vi "Old Limits Page.vi"(8 "error in (no error)":errorcluster, 10 "LBCB Number":T2) -> (0 "error out":errorcluster)   [LabVIEW 2013]
uses:
  lib/Limits/Faults List Actions.ctl
  lib/Limits Widget/Lower Upper Select.ctl
  lib/Limits Widget/Slider Messages.ctl
  lib/Data Access Objects/Metadata/LBCB Number.ctl
  lib/Control Loop/Parameter Change States.ctl
  lib/Control Loop/Parameters Changes.ctl
  lib/Data Access Objects/Application/Number Of LBCBs.ctl
  lib/Data Access Objects/Metadata/Persistant DAO Actions.ctl
  lib/Launcher/Launcher Actions.ctl
  lib/Launcher/NoPanelAppTypes.ctl
  lib/Logging/Debug Type.ctl
  lib/Limits Widget/Limits Page Visible Elements.ctl
  lib/Limits Widget/Limit Slider.ctl
  lib/Data Access Objects/Limits/DofTypes.ctl
panel:
  out "Messages":string
  in  "Ok":bool
  in  "DofType":T1
  in  "Limit Slider 6":T3
  in  "Limit Slider 5":T3
  in  "Limit Slider 4":T3
  in  "Limit Slider 3":T3
  in  "Limit Slider 2":T3
  in  "Limit Slider 1":T3
  # "Lower"
  # "Higher"
  # "Current"
  # "Lower"
  # "Higher"
  # "Current"
  # "Global"
  # "Local"
  # "Lower"
  # "Higher"
  # "Current"
  # "Lower"
  # "Higher"
  # "Current"
  # "Global"
  # "Local"
  # "Lower"
  # "Higher"
  # "Current"
  # "Lower"
  # "Higher"
  # "Current"
  # "Global"
  # "Local"
  # "Lower"
  # "Higher"
  # "Current"
  # "Lower"
  # "Higher"
  # "Current"
  # "Global"
  # "Local"
  # "Lower"
  # "Higher"
  # "Current"
  # "Lower"
  # "Higher"
  # "Current"
  # "Global"
  # "Local"
  # "Lower"
  # "Higher"
  # "Current"
  # "Lower"
  # "Higher"
  # "Current"
  # "Global"
  # "Local"
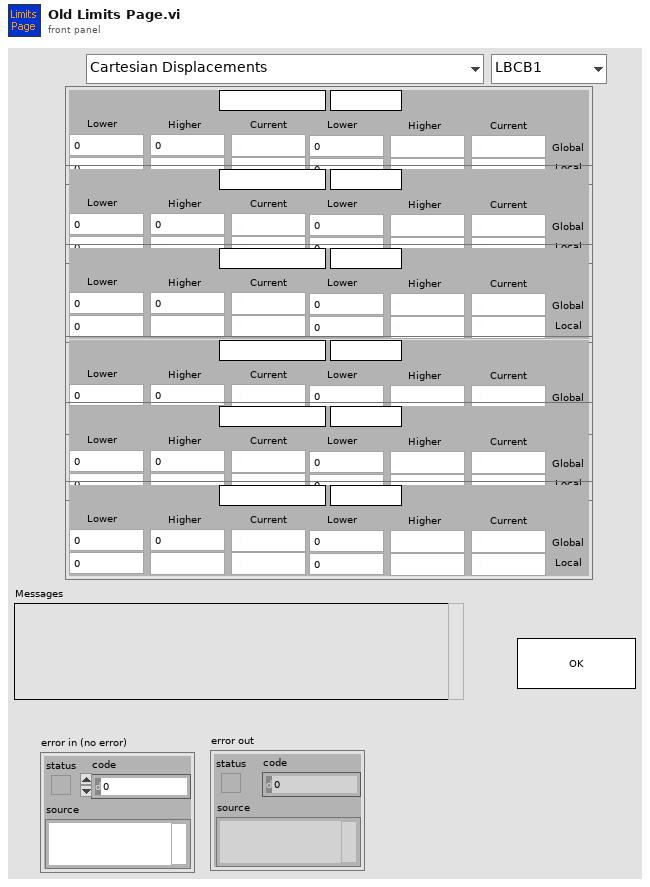
[diagram p1: front panel]
types:
  T1 = typedef "DofTypes.ctl" = enum16{"Cartesian Displacements", "Cartesian Forces & Moments", "Actuator Displacements", "Actuator Forces", "Cartesian Increments", "Actuator Increments"}
  T2 = typedef "LBCB Number.ctl" = enum16{"LBCB1", "LBCB2"}
  T3 = typedef "Limit Slider.ctl" = cluster{"DofLabel":string, "Units":string, "Global Lo 1":dbl, "Local Lo 1":dbl, "Global Hi 1":dbl, "Local Hi 1":dbl, "Global Actual 1":dbl, "Local Actual 1":dbl, "Global Lo 2":dbl, "Local Lo 2":dbl, "Global Hi 2":dbl, "Global Actual 2":dbl, "Local Hi 2":dbl, "Local Actual 2":dbl}
  T4 = typedef "Parameters Changes.ctl" = cluster{"Change State":T5, "LBCB Number":T2}
  T5 = typedef "Parameter Change States.ctl" = enum16{"Mixed Mode", "Control Loop", "Limits", "Application", "Stiffness Jacobian", "Start DAQ", "Reset Auto-Balance", "Set Command", "Enable Control", "Disable Control", "Position", "Stop Application"}
  T6 = typedef "Slider Messages.ctl" = enum16{"Update Display", "Exit", "Nothing"}
  T7 = typedef "Persistant DAO Actions.ctl" = enum16{"Init", "Get", "Set", "Load", "Save"}
  T8 = enum8{"Enabled", "Disabled", "Disabled and Grayed Out"}
  T9 = typedef "Number Of LBCBs.ctl" = enum16{"1", "2"}
  T10 = typedef "Faults List Actions.ctl" = enum16{"Init", "Add", "Remove", "Get List"}
  T11 = typedef "Lower Upper Select.ctl" = enum16{"Lower", "Upper"}
  T12 = typedef "Debug Type.ctl" = enum16{"Limit Update", "Limit Change", ""}
  T13 = typedef "Limits Page Visible Elements.ctl" = enum16{"All", "Global Only", "Low Only"}
  T14 = typedef "Fault Id.ctl" = cluster{"Fault Type":T15, "LBCB Number":T2, "Index":u32, "Space Type":T16}
  T15 = typedef "Fault Type.ctl" = enum16{"None", "Command", "Displacement", "Force", "Increment"}
  T16 = typedef "Space Type.ctl" = enum16{"Actuator", "Cartesian"}
  T17 = cluster{"[0]":dbl, "[1]":dbl, "[2]":dbl, "[3]":dbl, "[4]":dbl, "[5]":dbl, "[6]":dbl, "[7]":dbl, "[8]":dbl}[]
  T18 = cluster{"[0]":dbl, "[1]":dbl, "[2]":dbl, "[3]":dbl, "[4]":dbl, "[5]":dbl, "[6]":dbl, "[7]":dbl, "[8]":dbl}
  T19 = cluster{"[0]":dbl, "[1]":dbl, "[2]":dbl, "[3]":dbl}
  T20 = typedef "NoPanelAppTypes.ctl" = enum16{"NTCP Socket", "Data Archiving", "DAQ Link", "Control Loops", "Cmd Disp Diffs", "LBCB Data", "Limits", "Mixed Mode Widget", "Offsets", "Debug"}
  T21 = typedef "Launcher Actions.ctl" = enum16{"Launch", "Stop All", "Stop", "Kill", "Running?", "Init"}
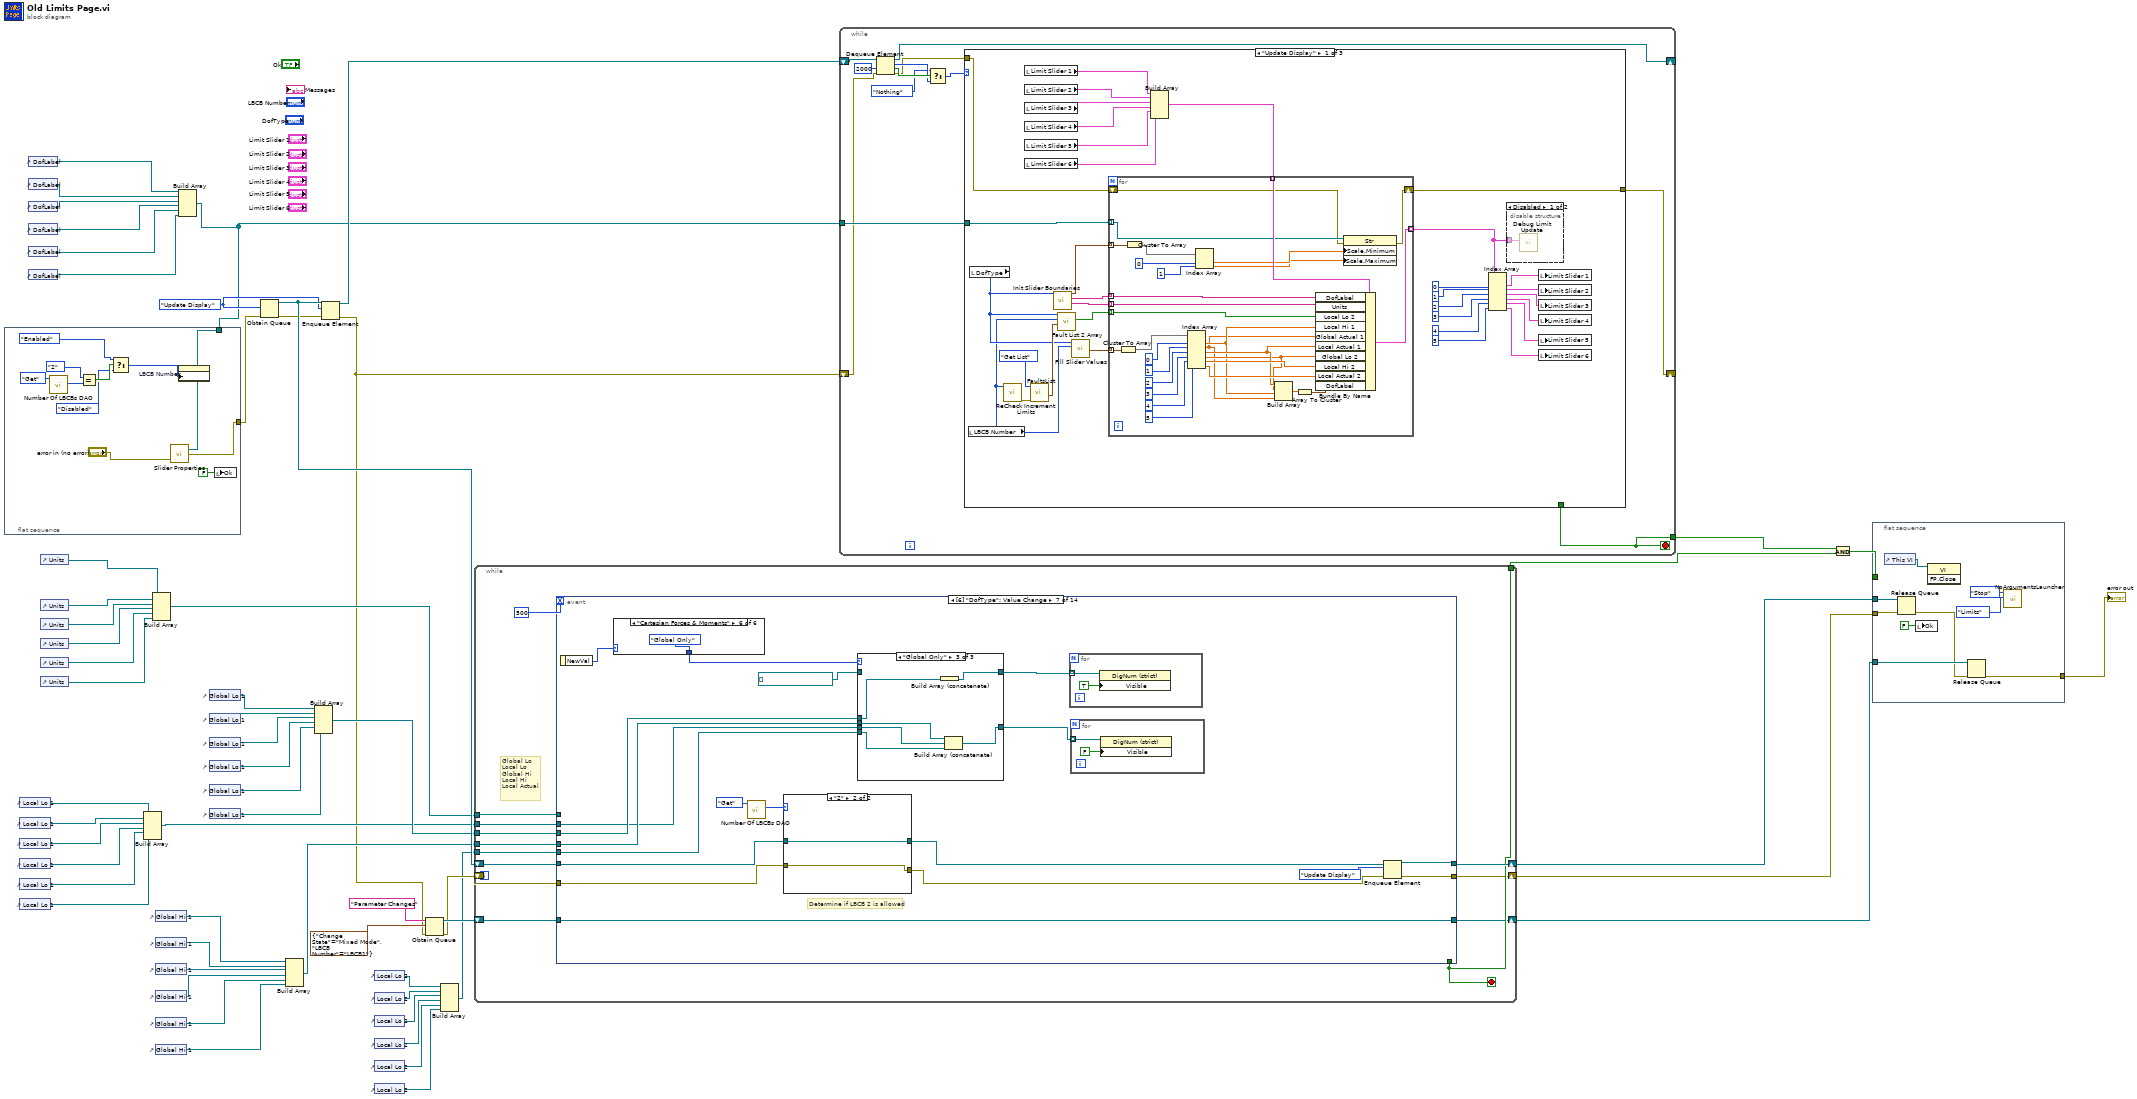
[diagram p0: block diagram]
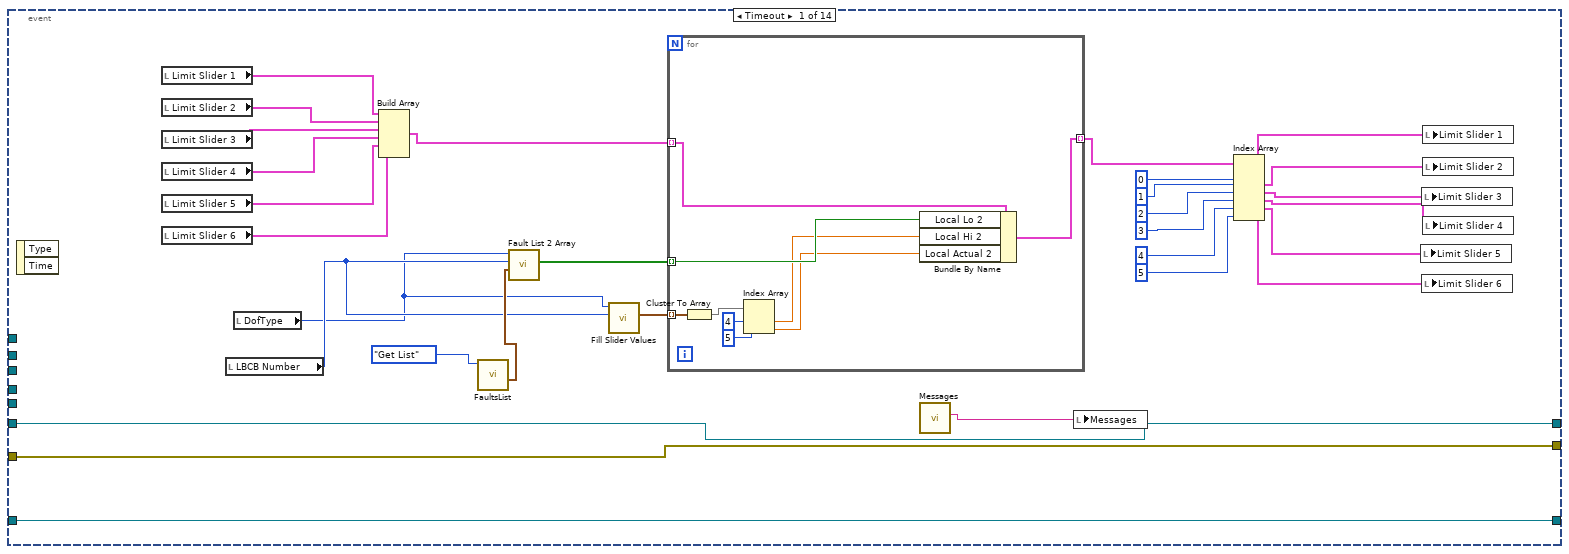
[diagram p2: hidden frame]
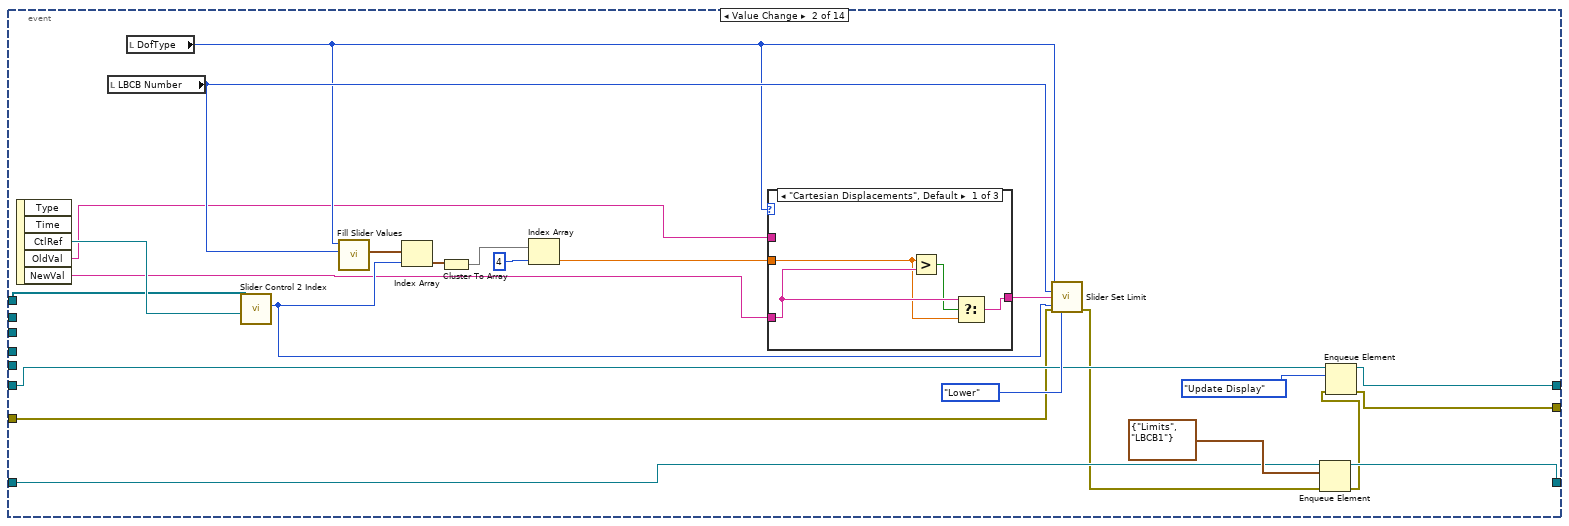
[diagram p3: hidden frame]
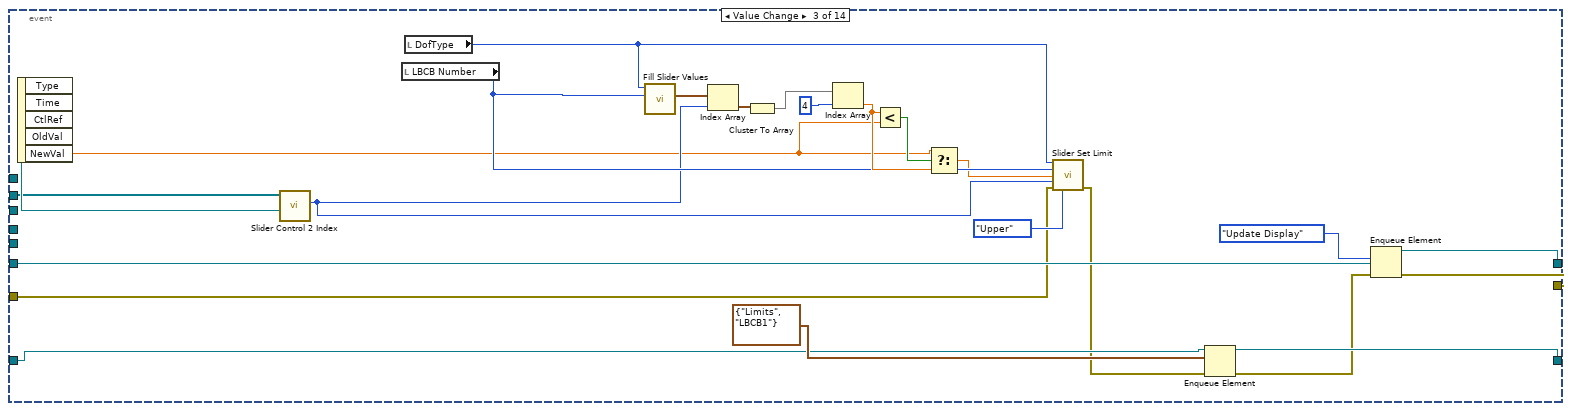
[diagram p6: hidden frame]
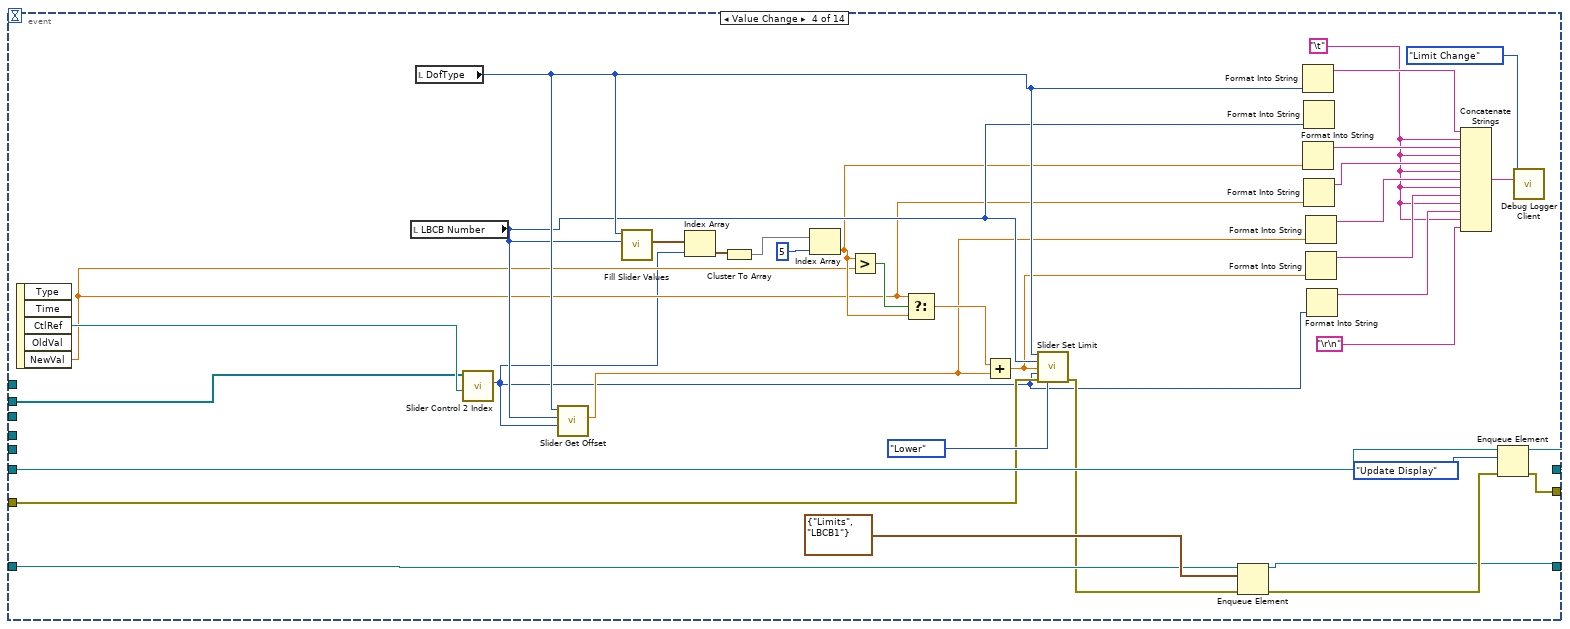
[diagram p7: hidden frame]
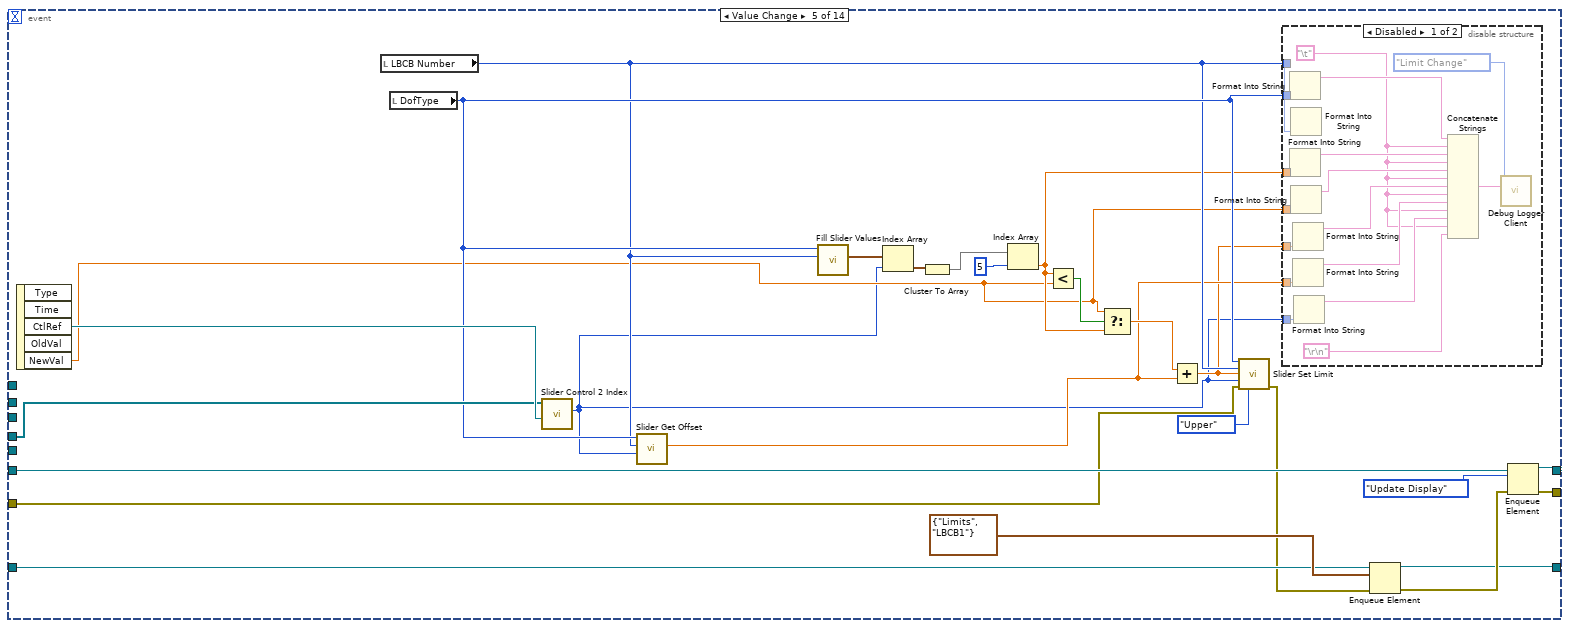
[diagram p8: hidden frame]
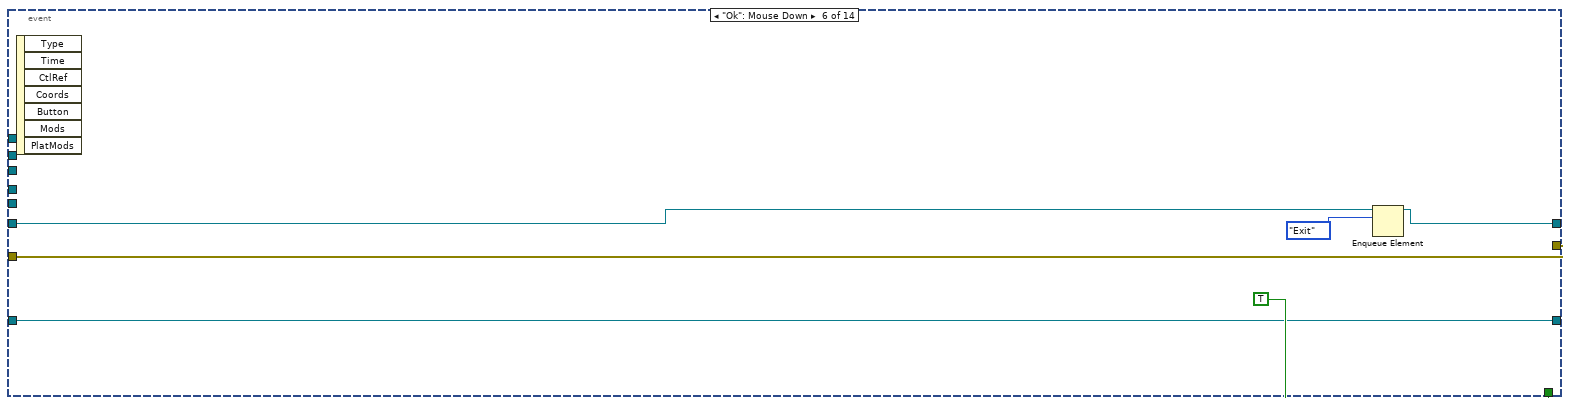
[diagram p10: hidden frame]
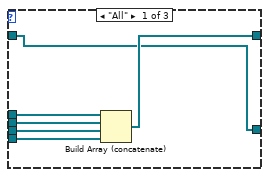
[diagram p11: hidden frame]
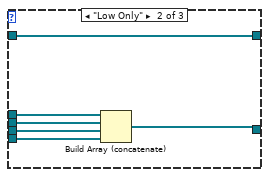
[diagram p12: hidden frame]
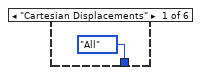
[diagram p13: hidden frame]
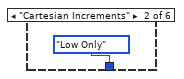
[diagram p14: hidden frame]
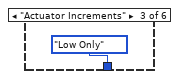
[diagram p15: hidden frame]
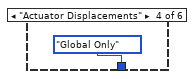
[diagram p16: hidden frame]
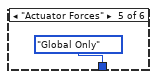
[diagram p17: hidden frame]
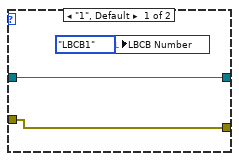
[diagram p18: hidden frame]
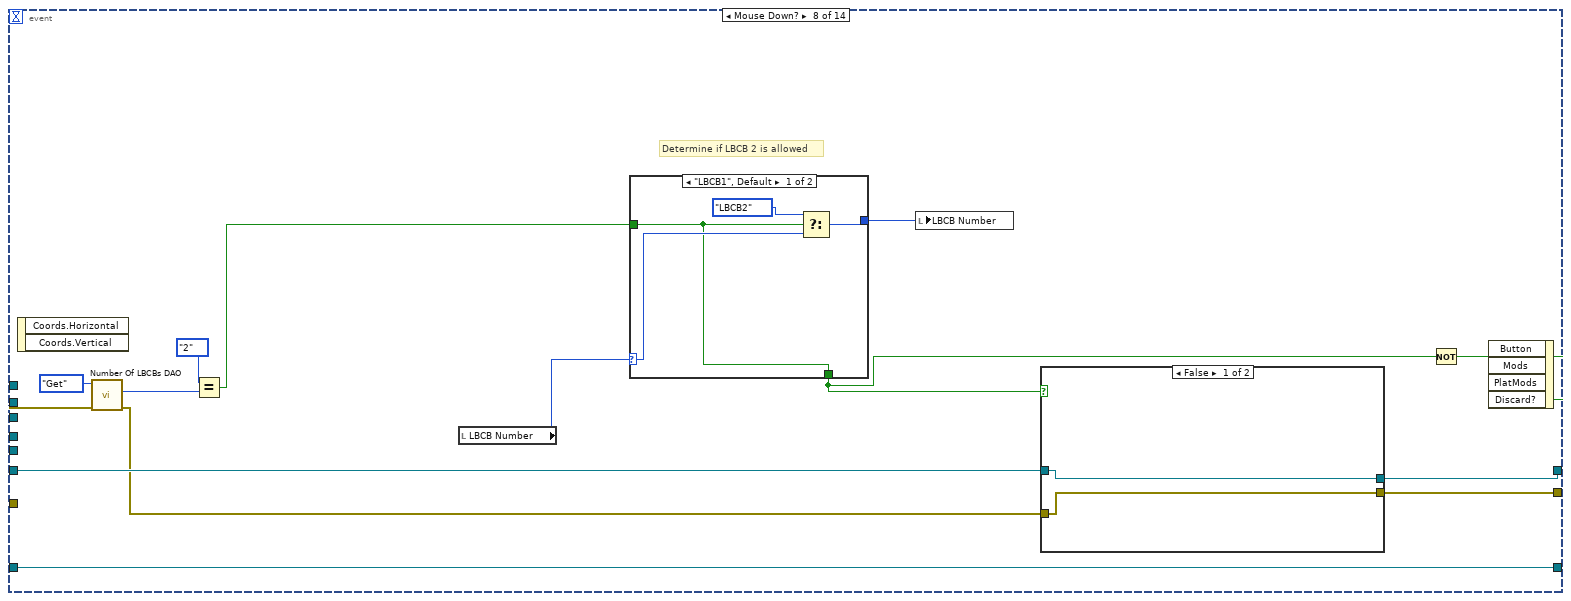
[diagram p19: hidden frame]
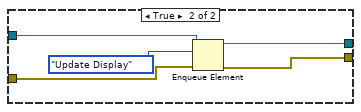
[diagram p20: hidden frame]
diagram:
  w54 = Slider_Messages."Update Display" ("Slider Message")
  n1 = flat-sequence {
    tunnel: w19 -> [w69]
    tunnel: [w68] -> w18
    frame #0 {
      n2 = call "Number Of LBCBs DAO.vi"("Actions"=Persistant_DAO_Actions."Get") -> ("Number of\nLBCBs Out"=w67:T9)  [unwired: 7 in, 3 out]
      n3 = Equal?(x=Number_Of_LBCBs."2", y=w67) -> (x = y?=w65:bool)
      n4 = Select(t=T8."Enabled" ("Disabled"), s=w65, f=T8."Disabled") -> (s? t:f=w62:T8)
      n5 = call "Slider Properties.vi"("error in (no error) 2"="error in (no error)", "Array"=w69) -> ("error out"=w68:errorcluster)
      n6 = property on="LBCB Number" class="Enum (strict)"("DisabledEnum"=w62) -> ()  [unwired: 2 in, 2 out]
      n7 = local write "Ok"(FALSE ("Ok")) -> ()
    }
  }
  n8 = control-ref of="Local Lo 1"() -> (w41:refnum<vi>)
  n9 = control-ref of="Local Lo 1"() -> (w40:refnum<vi>)
  n10 = control-ref of="Local Lo 1"() -> (w39:refnum<vi>)
  n11 = control-ref of="Local Lo 1"() -> (w38:refnum<vi>)
  n12 = control-ref of="Local Lo 1"() -> (w37:refnum<vi>)
  n13 = control-ref of="Local Lo 1"() -> (w36:refnum<vi>)
  n14 = control-ref of="DofLabel"() -> (w53:refnum<vi>)
  n15 = control-ref of="DofLabel"() -> (w52:refnum<vi>)
  n16 = control-ref of="DofLabel"() -> (w51:refnum<vi>)
  n17 = control-ref of="DofLabel"() -> (w50:refnum<vi>)
  n18 = control-ref of="DofLabel"() -> (w49:refnum<vi>)
  n19 = control-ref of="DofLabel"() -> (w48:refnum<vi>)
  n20 = control-ref of="Units"() -> (w47:refnum<vi>)
  n21 = control-ref of="Units"() -> (w46:refnum<vi>)
  n22 = control-ref of="Units"() -> (w45:refnum<vi>)
  n23 = control-ref of="Units"() -> (w44:refnum<vi>)
  n24 = control-ref of="Units"() -> (w43:refnum<vi>)
  n25 = control-ref of="Units"() -> (w42:refnum<vi>)
  n26 = Build Array(w41, w40, w39, w38, w37, w36) -> (w22:refnum<vi>[])
  n27 = Build Array(w47, w46, w45, w44, w43, w42) -> (w21:refnum<vi>[])
  n28 = control-ref of="Global Hi 1"() -> (w29:refnum<vi>)
  n29 = control-ref of="Global Hi 1"() -> (w28:refnum<vi>)
  n30 = control-ref of="Global Hi 1"() -> (w16:refnum<vi>)
  n31 = control-ref of="Global Hi 1"() -> (w27:refnum<vi>)
  n32 = control-ref of="Global Hi 1"() -> (w26:refnum<vi>)
  n33 = control-ref of="Global Hi 1"() -> (w25:refnum<vi>)
  n34 = Build Array(w53, w52, w51, w50, w49, w48) -> (w19:refnum<vi>[])
  n35 = control-ref of="Global Lo 1"() -> (w35:refnum<vi>)
  n36 = control-ref of="Global Lo 1"() -> (w34:refnum<vi>)
  n37 = control-ref of="Global Lo 1"() -> (w33:refnum<vi>)
  n38 = control-ref of="Global Lo 1"() -> (w32:refnum<vi>)
  n39 = control-ref of="Global Lo 1"() -> (w31:refnum<vi>)
  n40 = control-ref of="Global Lo 1"() -> (w30:refnum<vi>)
  n41 = Obtain Queue(element data type=w54, error in (no error)=w18) -> (queue out=w59:refnum<queue>, error out=w20:errorcluster)  [unwired: 3 in, 1 out]
  n42 = Build Array(w29, w28, w16, w27, w26, w25) -> (w24:refnum<vi>[])
  n43 = Build Array(w35, w34, w33, w32, w31, w30) -> (w23:refnum<vi>[])
  n44 = Enqueue Element(queue=w59, element=w54, error in (no error)=w20) -> (queue out=w55:refnum<queue>, error out=w12:errorcluster)  [unwired: 1 in, 1 out]
  n45 = control-ref of="Local Lo 2"() -> (w7:refnum<vi>)
  n46 = control-ref of="Local Lo 2"() -> (w6:refnum<vi>)
  n47 = control-ref of="Local Lo 2"() -> (w5:refnum<vi>)
  n48 = control-ref of="Local Lo 2"() -> (w4:refnum<vi>)
  n49 = control-ref of="Local Lo 2"() -> (w3:refnum<vi>)
  n50 = control-ref of="Local Lo 2"() -> (w2:refnum<vi>)
  n51 = Obtain Queue(name (unnamed)="Parameter Changes", element data type=T4 {"Change State"=enum."Mixed Mode", "LBCB Number"=enum."LBCB1"} ("Parameter Changes"), error in (no error)=w12) -> (queue out=w13:refnum<queue>, error out=w11:errorcluster)  [unwired: 2 in, 1 out]
  n52 = Build Array(w7, w6, w5, w4, w3, w2) -> (w1:refnum<vi>[])
  n53 = while {
    shift-right: [w82] -> w17
    shift-left: w59 -> [w83]
    tunnel: [w81] -> w57
    tunnel: w24 -> [w78]
    tunnel: w23 -> [w77]
    tunnel: w22 -> [w79]
    tunnel: w21 -> [w80]
    shift-right: [w75] -> w9
    shift-left: w11 -> [w76]
    shift-right: [w73] -> w10
    shift-left: w13 -> [w74]
    tunnel: w1 -> [w72]
    stop <- w81 stop-if-true
    # "Global Lo\nLocal Lo\nGlobal Hi\nLocal Hi\nLocal Actual"
    n54 = event shown="[6] \"DofType\": Value Change" {
      selector: _ -> [_ _ _ _ _ _ _ _ _ _ _ _ _ _]
      dyn-events: _ -> [_ _ _ _ _ _ _ _ _ _ _ _ _ _]
      timeout: 500 -> [_ _ _ _ _ _ _ _ _ _ _ _ _ _]
      tunnel: w83 -> [w112 w143 w173 w209 w236 w260 w275 w327 w348 w397 w446 w497 w544 w593]
      tunnel: [w112 w142 w172 w208 w234 w259 w279 w326 w347 w396 w445 w496 w543 w592] -> w82
      tunnel: [_ _ _ _ _ TRUE _ _ _ _ _ _ _ _] -> w81
      tunnel: w80 -> [_ w141 _ _ _ _ _ _ _ _ _ _ _ _]
      tunnel: w79 -> [_ _ _ w207 _ _ w266 _ _ _ _ _ _ _]
      tunnel: w78 -> [_ _ _ _ w233 _ w268 _ _ _ _ _ _ _]
      tunnel: w77 -> [_ _ w171 _ _ _ w269 _ _ _ _ _ _ _]
      tunnel: w76 -> [w111 w140 w170 w206 w232 w257 w273 w323 w350 w399 w448 w499 w546 w595]
      tunnel: [w111 w139 w169 w205 w231 w257 w278 w325 w346 w395 w444 w495 w542 w591] -> w75
      tunnel: w74 -> [w110 w137 w167 w203 w229 w256 w277 w324 w344 w393 w442 w491 w540 w589]
      tunnel: [w110 w136 w166 w200 w226 w256 w277 w324 w343 w392 w440 w490 w539 w588] -> w73
      tunnel: w72 -> [_ _ _ _ _ _ w265 _ _ _ _ _ _ _]
      event Timeout {
        n55 = event-data() -> ()  [unwired: 1 in, 2 out]
        n56 = local read "Limit Slider 1"() -> (w107:T3)
        n57 = local read "Limit Slider 2"() -> (w106:T3)
        n58 = local read "Limit Slider 3"() -> (w105:T3)
        n59 = local read "Limit Slider 4"() -> (w104:T3)
        n60 = local read "Limit Slider 5"() -> (w103:T3)
        n61 = local read "Limit Slider 6"() -> (w102:T3)
        n62 = local read "LBCB Number"() -> (w86:T2)
        n63 = local read "DofType"() -> (w85:T1)
        n64 = Build Array(w107, w106, w105, w104, w103, w102) -> (w94:T3[])
        n65 = call "FaultsList.vi"("Limits List Actions"=Faults_List_Actions."Get List") -> ("Fault List"=w108:T14[])  [unwired: 2 in, 8 out]
        n66 = call "Fault List 2 Array.vi"("Fault List"=w108, "LBCB Number"=w86, "DofType"=w85) -> ("Faults"=w95:bool[])  [unwired: 8 in]
        n67 = call "Fill Slider Values.vi"("LBCB Number"=w86, "DofType"=w85) -> ("Silder Values"=w84:T17)  [unwired: 9 in]
        n68 = for {
          tunnel: w95 -> [w121] mode=indexing
          tunnel: w94 -> [w122] mode=indexing
          tunnel: [w120] -> w93 mode=indexing
          tunnel: w84 -> [w119] mode=indexing
          n69 = Cluster To Array(cluster=w119) -> (array=w118:dbl[])
          n70 = Index Array(array=w118, index #1=4 ("index"), index #2=5 ("index")) -> (element #1=w115:dbl, element #2=w114:dbl)
          n71 = Bundle By Name(cluster=w122, "Local Lo 2"=w121, "Local Hi 2"=w115, "Local Actual 2"=w114) -> (w120:T3)
        }
        n72 = call "Messages.vi"() -> ("Messages"=w113:string)  [unwired: 2 in, 9 out]
        n73 = local write "Messages"(w113) -> ()
        n74 = Index Array(array=w93, index #1=0 ("index"), index #2=1 ("index"), index #3=2 ("index"), index #4=3 ("index"), index #5=4 ("index"), index #6=5 ("index")) -> (element #1=w92:T3, element #2=w91:T3, element #3=w90:T3, element #4=w89:T3, element #5=w88:T3, element #6=w87:T3)
        n75 = local write "Limit Slider 5"(w88) -> ()
        n76 = local write "Limit Slider 3"(w90) -> ()
        n77 = local write "Limit Slider 6"(w87) -> ()
        n78 = local write "Limit Slider 1"(w92) -> ()
        n79 = local write "Limit Slider 2"(w91) -> ()
        n80 = local write "Limit Slider 4"(w89) -> ()
      }
      event Value Change {
        n81 = event-data() -> ("CtlRef"=w146:refnum<vi>, "OldVal"=w123:string, "NewVal"=w127:string)  [unwired: 1 in, 2 out]
        n82 = local read "LBCB Number"() -> (w133:T2)
        n83 = local read "DofType"() -> (w124:T1)
        n84 = call "Slider Control 2 Index.vi"("Control"=w146, "Controls"=w141) -> ("Index"=w131:i32)  [unwired: 9 in]
        n85 = call "Fill Slider Values.vi"("LBCB Number"=w133, "DofType"=w124) -> ("Silder Values"=w132:T17)  [unwired: 9 in]
        n86 = Index Array(array=w132, index=w131) -> (element=w130:T18)
        n87 = Cluster To Array(cluster=w130) -> (array=w129:dbl[])
        n88 = Index Array(array=w129, index=4) -> (element=w125:dbl)
        n89 = case shown="\"Cartesian Displacements\", Default" w124 {
          tunnel: w127 -> [w150 w151 w152]
          tunnel: [w149 w151 w152] -> w126
          tunnel: w125 -> [w147 _ _]
          tunnel: w123 -> [_ _ _]
          frame "Cartesian Displacements", Default {
            n90 = Greater?(x=w147, y=w150) -> (0:w148:bool)
            n91 = Select(t=w150, s=w148, f=w147) -> (s? t:f=w149:string)
          }
          frame "Cartesian Increments" {
          }
          frame "Actuator Increments" {
          }
        }
        n92 = call "Slider Set Limit.vi"("DofType"=w124, "LBCB Number"=w133, "Value"=w126, "Index"=w131, "error in (no error)"=w140, "Lower/Upper"=Lower_Upper_Select."Lower") -> ("error out"=w135:errorcluster)  [unwired: 9 in]
        n93 = Enqueue Element(queue=w137, element=T4 {"Change State"=enum."Limits", "LBCB Number"=enum."LBCB1"}, error in (no error)=w135) -> (queue out=w136:refnum<queue>, error out=w134:errorcluster)  [unwired: 2 out]
        n94 = Enqueue Element(queue=w143, element=Slider_Messages."Update Display", error in (no error)=w134) -> (queue out=w142:refnum<queue>, error out=w139:errorcluster)  [unwired: 1 in, 1 out]
      }
      event Value Change {
        n95 = event-data() -> ("CtlRef"=w176:refnum<vi>, "NewVal"=w153:dbl)  [unwired: 1 in, 3 out]
        n96 = call "Slider Control 2 Index.vi"("Control"=w176, "Controls"=w171) -> ("Index"=w155:i32)  [unwired: 9 in]
        n97 = local read "LBCB Number"() -> (w156:T2)
        n98 = local read "DofType"() -> (w157:T1)
        n99 = call "Fill Slider Values.vi"("LBCB Number"=w156, "DofType"=w157) -> ("Silder Values"=w163:T17)  [unwired: 9 in]
        n100 = Index Array(array=w163, index=w155) -> (element=w162:T18)
        n101 = Cluster To Array(cluster=w162) -> (array=w161:dbl[])
        n102 = Index Array(array=w161, index=4) -> (element=w158:dbl)
        n103 = Less?(x=w158, y=w153) -> (x < y?=w159:bool)
        n104 = Select(t=w153, s=w159, f=w158) -> (s? t:f=w154:dbl)
        n105 = call "Slider Set Limit.vi"("DofType"=w157, "LBCB Number"=w156, "Value"=w154, "Index"=w155, "error in (no error)"=w170, "Lower/Upper"=Lower_Upper_Select."Upper") -> ("error out"=w165:errorcluster)  [unwired: 9 in]
        n106 = Enqueue Element(queue=w167, element=T4 {"Change State"=enum."Limits", "LBCB Number"=enum."LBCB1"}, error in (no error)=w165) -> (queue out=w166:refnum<queue>, error out=w164:errorcluster)  [unwired: 2 out]
        n107 = Enqueue Element(queue=w173, element=Slider_Messages."Update Display", error in (no error)=w164) -> (queue out=w172:refnum<queue>, error out=w169:errorcluster)  [unwired: 1 in, 1 out]
      }
      event Value Change {
        w187 = "\t"
        n108 = event-data() -> ("CtlRef"=w212:refnum<vi>, "NewVal"=w180:dbl)  [unwired: 1 in, 3 out]
        n109 = local read "LBCB Number"() -> (w182:T2)
        n110 = local read "DofType"() -> (w183:T1)
        n111 = call "Slider Control 2 Index.vi"("Control"=w212, "Controls"=w207) -> ("Index"=w177:i32)  [unwired: 9 in]
        n112 = call "Slider Get Offset.vi"("Index"=w177, "LBCB Number"=w182, "DofType"=w183) -> ("Offset"=w179:dbl)  [unwired: 8 in]
        n113 = call "Fill Slider Values.vi"("LBCB Number"=w182, "DofType"=w183) -> ("Silder Values"=w199:T17)  [unwired: 9 in]
        n114 = Index Array(array=w199, index=w177) -> (element=w198:T18)
        n115 = Cluster To Array(cluster=w198) -> (array=w197:dbl[])
        n116 = Index Array(array=w197, index=5) -> (element=w181:dbl)
        n117 = Greater?(x=w181, y=w180) -> (0:w195:bool)
        n118 = Select(t=w180, s=w195, f=w181) -> (s? t:f=w194:dbl)
        n119 = Add(x=w194, y=w179) -> (x+y=w178:dbl)
        n120 = call "Slider Set Limit.vi"("DofType"=w183, "LBCB Number"=w182, "Value"=w178, "Index"=w177, "error in (no error)"=w206, "Lower/Upper"=Lower_Upper_Select."Lower") -> ("error out"=w202:errorcluster)  [unwired: 9 in]
        n121 = Enqueue Element(queue=w203, element=T4 {"Change State"=enum."Limits", "LBCB Number"=enum."LBCB1"}, error in (no error)=w202) -> (queue out=w200:refnum<queue>, error out=w201:errorcluster)  [unwired: 2 out]
        n122 = Format Into String(w183) -> (resulting string=w193:string)  [unwired: 3 in, 1 out]
        n123 = Format Into String(w181) -> (resulting string=w192:string)  [unwired: 3 in, 1 out]
        n124 = Format Into String(w182) -> ()  [unwired: 3 in, 2 out]
        n125 = Format Into String(w180) -> (resulting string=w191:string)  [unwired: 3 in, 1 out]
        n126 = Format Into String(w179) -> (resulting string=w190:string)  [unwired: 3 in, 1 out]
        n127 = Format Into String(w178) -> (resulting string=w189:string)  [unwired: 3 in, 1 out]
        n128 = Format Into String(w177) -> (resulting string=w188:string)  [unwired: 3 in, 1 out]
        n129 = Concatenate Strings(w193, w187, w192, w187, w191, w187, w190, w187, w189, w187, w188, w187, "\r\n") -> (w185:string)
        n130 = Enqueue Element(queue=w209, element=Slider_Messages."Update Display", error in (no error)=w201) -> (queue out=w208:refnum<queue>, error out=w205:errorcluster)  [unwired: 1 in, 1 out]
        n131 = call "Debug Logger Client.vi"("Message"=w185, "Debug Type"=Debug_Type."Limit Change") -> ()  [unwired: 9 in, 1 out]
      }
      event Value Change {
        n132 = event-data() -> ("CtlRef"=w238:refnum<vi>, "NewVal"=w217:dbl)  [unwired: 1 in, 3 out]
        n133 = local read "LBCB Number"() -> (w219:T2)
        n134 = local read "DofType"() -> (w220:T1)
        n135 = call "Slider Control 2 Index.vi"("Control"=w238, "Controls"=w233) -> ("Index"=w213:i32)  [unwired: 9 in]
        n136 = call "Slider Get Offset.vi"("Index"=w213, "LBCB Number"=w219, "DofType"=w220) -> ("Offset"=w215:dbl)  [unwired: 8 in]
        n137 = call "Fill Slider Values.vi"("LBCB Number"=w219, "DofType"=w220) -> ("Silder Values"=w225:T17)  [unwired: 9 in]
        n138 = Index Array(array=w225, index=w213) -> (element=w224:T18)
        n139 = Cluster To Array(cluster=w224) -> (array=w223:dbl[])
        n140 = Index Array(array=w223, index=5) -> (element=w218:dbl)
        n141 = Less?(x=w218, y=w217) -> (x < y?=w221:bool)
        n142 = Select(t=w217, s=w221, f=w218) -> (s? t:f=w216:dbl)
        n143 = Add(x=w216, y=w215) -> (x+y=w214:dbl)
        n144 = call "Slider Set Limit.vi"("DofType"=w220, "LBCB Number"=w219, "Value"=w214, "Index"=w213, "error in (no error)"=w232, "Lower/Upper"=Lower_Upper_Select."Upper") -> ("error out"=w228:errorcluster)  [unwired: 9 in]
        n145 = disable-structure shown="Disabled" {
          disable-tunnel: w220 -> [w255 _]
          disable-tunnel: w219 -> [w254 _]
          disable-tunnel: w218 -> [w253 _]
          disable-tunnel: w217 -> [w252 _]
          disable-tunnel: w215 -> [w251 _]
          disable-tunnel: w214 -> [w250 _]
          disable-tunnel: w213 -> [w249 _]
          frame Disabled {
            w242 = "\t"
            n146 = Format Into String(w255) -> (resulting string=w248:string)  [unwired: 3 in, 1 out]
            n147 = Format Into String(w253) -> (resulting string=w247:string)  [unwired: 3 in, 1 out]
            n148 = Format Into String(w254) -> ()  [unwired: 3 in, 2 out]
            n149 = Format Into String(w252) -> (resulting string=w246:string)  [unwired: 3 in, 1 out]
            n150 = Format Into String(w250) -> (resulting string=w245:string)  [unwired: 3 in, 1 out]
            n151 = Format Into String(w251) -> (resulting string=w244:string)  [unwired: 3 in, 1 out]
            n152 = Format Into String(w249) -> (resulting string=w243:string)  [unwired: 3 in, 1 out]
            n153 = Concatenate Strings(w248, w242, w247, w242, w246, w242, w245, w242, w244, w242, w243, w242, "\r\n") -> (w240:string)
            n154 = call "Debug Logger Client.vi"("Message"=w240, "Debug Type"=Debug_Type."Limit Change") -> ()  [unwired: 9 in, 1 out]
          }
          frame Enabled {
          }
        }
        n155 = Enqueue Element(queue=w229, element=T4 {"Change State"=enum."Limits", "LBCB Number"=enum."LBCB1"}, error in (no error)=w228) -> (queue out=w226:refnum<queue>, error out=w227:errorcluster)  [unwired: 2 out]
        n156 = Enqueue Element(queue=w236, element=Slider_Messages."Update Display", error in (no error)=w227) -> (queue out=w234:refnum<queue>, error out=w231:errorcluster)  [unwired: 1 in, 1 out]
      }
      event "Ok": Mouse Down {
        n157 = event-data() -> ()  [unwired: 1 in, 7 out]
        n158 = Enqueue Element(queue=w260, element=Slider_Messages."Exit") -> (queue out=w259:refnum<queue>)  [unwired: 2 in, 2 out]
      }
      event Value Change {
        # "Determine if LBCB 2 is allowed"
        n159 = event-data() -> ("NewVal"=w270:T1)  [unwired: 1 in]
        n160 = case shown="\"Cartesian Forces & Moments\"" w270 {
          tunnel: [Limits_Page_Visible_Elements."All" ("Limits Page Visible Elements") Limits_Page_Visible_Elements."Low Only" ("Limits Page Visible Elements") Limits_Page_Visible_Elements."Low Only" ("Limits Page Visible Elements") Limits_Page_Visible_Elements."Global Only" ("Limits Page Visible Elements") Limits_Page_Visible_Elements."Global Only" ("Limits Page Visible Elements") Limits_Page_Visible_Elements."Global Only" ("Limits Page Visible Elements")] -> w264
          frame "Cartesian Displacements" {
          }
          frame "Cartesian Increments" {
          }
          frame "Actuator Increments" {
          }
          frame "Actuator Displacements" {
          }
          frame "Actuator Forces" {
          }
          frame "Cartesian Forces & Moments" {
          }
        }
        n161 = call "Number Of LBCBs DAO.vi"("Actions"=Persistant_DAO_Actions."Get") -> ("Number of\nLBCBs Out"=w271:T9)  [unwired: 7 in, 3 out]
        n162 = case shown="\"2\"" w271 {
          tunnel: w275 -> [w311 w313]
          tunnel: [w311 w313] -> w274
          tunnel: w273 -> [w310 w312]
          tunnel: [w310 w312] -> w272
          frame "1", Default {
            n163 = local write "LBCB Number"(LBCB_Number."LBCB1" ("LBCB Number")) -> ()
          }
          frame "2" {
          }
        }
        n164 = case shown="\"Global Only\"" w264 {
          tunnel: w269 -> [w288 w294 w296]
          tunnel: w268 -> [w287 w293 w295]
          tunnel: [w286 w289 w298] -> w267
          tunnel: w266 -> [w285 w292 w300]
          tunnel: w265 -> [w284 w291 w299]
          tunnel: [w283 w290 w297] -> w263
          tunnel: refnum<vi>[] [] -> [w283 w289 _]
          frame "All" {
            n165 = Build Array (concatenate)(w288, w287, w285, w284) -> (w286:refnum<vi>[])
          }
          frame "Low Only" {
            n166 = Build Array (concatenate)(w294, w293, w292, w291) -> (w290:refnum<vi>[])
          }
          frame "Global Only" {
            n167 = Build Array (concatenate)(w296) -> (w298:refnum<vi>[])
            n168 = Build Array (concatenate)(w295, w300, w299) -> (w297:refnum<vi>[])
          }
        }
        n169 = for {
          tunnel: w267 -> [w302] mode=indexing
          n170 = property class="DigNum (strict)"(reference=w302, "Visible"=TRUE) -> ()  [unwired: 1 in, 2 out]
        }
        n171 = for {
          tunnel: w263 -> [w282] mode=indexing
          n172 = property class="DigNum (strict)"(reference=w282, "Visible"=FALSE) -> ()  [unwired: 1 in, 2 out]
        }
        n173 = Enqueue Element(queue=w274, element=Slider_Messages."Update Display", error in (no error)=w272) -> (queue out=w279:refnum<queue>, error out=w278:errorcluster)  [unwired: 1 in, 1 out]
      }
      event Mouse Down? {
        # "Determine if LBCB 2 is allowed"
        n174 = event-data() -> ()  [unwired: 1 in, 2 out]
        n175 = call "Number Of LBCBs DAO.vi"("error in (no error)"=w323, "Actions"=Persistant_DAO_Actions."Get") -> ("error out"=w321:errorcluster, "Number of\nLBCBs Out"=w320:T9)  [unwired: 6 in, 2 out]
        n176 = Equal?(x=Number_Of_LBCBs."2", y=w320) -> (x = y?=w314:bool)
        n177 = local read "LBCB Number"() -> (w318:T2)
        n178 = case shown="\"LBCB1\", Default" w318 {
          selector: w318 -> [w337 _]
          tunnel: [w338 LBCB_Number."LBCB1" ("LBCB Number")] -> w317
          tunnel: w314 -> [w335 _]
          tunnel: [w335 TRUE] -> w316
          frame "LBCB1", Default {
            n179 = Select(t=LBCB_Number."LBCB2", s=w335, f=w337) -> (s? t:f=w338:T2)
          }
          frame "LBCB2" {
          }
        }
        n180 = local write "LBCB Number"(w317) -> ()
        n181 = case shown="False" w316 {
          tunnel: w327 -> [w329 w334]
          tunnel: [w329 w333] -> w326
          tunnel: [w328 w332] -> w325
          tunnel: w321 -> [w328 w331]
          frame False {
          }
          frame True {
            n182 = Enqueue Element(queue=w334, element=Slider_Messages."Update Display", error in (no error)=w331) -> (queue out=w333:refnum<queue>, error out=w332:errorcluster)  [unwired: 1 in, 1 out]
          }
        }
        n183 = Not(x=w316) -> (.not. x?=w315:bool)
        n184 = event-data("Discard?"=w315) -> ()  [unwired: 4 in, 1 out]
      }
      event Value Change {
        n185 = event-data() -> ("OldVal"=w357:string, "NewVal"=w356:string)  [unwired: 1 in, 3 out]
        n186 = call "Limit Crossover Check.vi"("NewVal"=w356, "OldVal"=w357) -> ("Value"=w352:dbl, "Index"=w353:i32)
        n187 = local read "LBCB Number"() -> (w354:T2)
        n188 = local read "DofType"() -> (w355:T1)
        n189 = case shown="0, Default" w353 {
          tunnel: w355 -> [w366 w375 w382 w389]
          tunnel: w354 -> [w365 w374 w381 w388]
          tunnel: w352 -> [w362 w371 w376 w383]
          tunnel: 0 ("Index") -> [w364 w373 w380 w387]
          tunnel: w350 -> [w360 w369 w379 w386]
          tunnel: [w359 w368 w378 w385] -> w342
          frame 0, Default {
            n190 = call "Slider Get Offset.vi"("Index"=w364, "LBCB Number"=w365, "DofType"=w366) -> ("Offset"=w361:dbl)  [unwired: 8 in]
            n191 = Add(x=w362, y=w361) -> (x+y=w363:dbl)
            n192 = call "Slider Set Limit.vi"("DofType"=w366, "LBCB Number"=w365, "Value"=w363, "Index"=w364, "error in (no error)"=w360, "Lower/Upper"=Lower_Upper_Select."Lower") -> ("error out"=w359:errorcluster)  [unwired: 9 in]
          }
          frame 1 {
            n193 = call "Slider Get Offset.vi"("Index"=w373, "LBCB Number"=w374, "DofType"=w375) -> ("Offset"=w370:dbl)  [unwired: 8 in]
            n194 = Add(x=w371, y=w370) -> (x+y=w372:dbl)
            n195 = call "Slider Set Limit.vi"("DofType"=w375, "LBCB Number"=w374, "Value"=w372, "Index"=w373, "error in (no error)"=w369, "Lower/Upper"=Lower_Upper_Select."Upper") -> ("error out"=w368:errorcluster)  [unwired: 9 in]
          }
          frame 2 {
            n196 = call "Slider Set Limit.vi"("DofType"=w382, "LBCB Number"=w381, "Value"=w376, "Index"=w380, "error in (no error)"=w379, "Lower/Upper"=Lower_Upper_Select."Lower") -> ("error out"=w378:errorcluster)  [unwired: 9 in]
          }
          frame 3 {
            n197 = call "Slider Set Limit.vi"("DofType"=w389, "LBCB Number"=w388, "Value"=w383, "Index"=w387, "error in (no error)"=w386, "Lower/Upper"=Lower_Upper_Select."Upper") -> ("error out"=w385:errorcluster)  [unwired: 9 in]
          }
        }
        n198 = Enqueue Element(queue=w344, element=T4 {"Change State"=enum."Limits", "LBCB Number"=enum."LBCB1"}, error in (no error)=w342) -> (queue out=w343:refnum<queue>, error out=w341:errorcluster)  [unwired: 2 out]
        n199 = Enqueue Element(queue=w348, element=Slider_Messages."Update Display", error in (no error)=w341) -> (queue out=w347:refnum<queue>, error out=w346:errorcluster)  [unwired: 1 in, 1 out]
      }
      event Value Change {
        n200 = event-data() -> ("OldVal"=w406:string, "NewVal"=w405:string)  [unwired: 1 in, 3 out]
        n201 = local read "LBCB Number"() -> (w403:T2)
        n202 = call "Limit Crossover Check.vi"("NewVal"=w405, "OldVal"=w406) -> ("Value"=w401:dbl, "Index"=w402:i32)
        n203 = local read "DofType"() -> (w404:T1)
        n204 = case shown="0, Default" w402 {
          tunnel: w404 -> [w415 w424 w431 w438]
          tunnel: w403 -> [w414 w423 w430 w437]
          tunnel: w401 -> [w411 w420 w425 w432]
          tunnel: 1 ("Index") -> [w413 w422 w429 w436]
          tunnel: w399 -> [w409 w418 w428 w435]
          tunnel: [w408 w417 w427 w434] -> w391
          frame 0, Default {
            n205 = call "Slider Get Offset.vi"("Index"=w413, "LBCB Number"=w414, "DofType"=w415) -> ("Offset"=w410:dbl)  [unwired: 8 in]
            n206 = Add(x=w411, y=w410) -> (x+y=w412:dbl)
            n207 = call "Slider Set Limit.vi"("DofType"=w415, "LBCB Number"=w414, "Value"=w412, "Index"=w413, "error in (no error)"=w409, "Lower/Upper"=Lower_Upper_Select."Lower") -> ("error out"=w408:errorcluster)  [unwired: 9 in]
          }
          frame 1 {
            n208 = call "Slider Get Offset.vi"("Index"=w422, "LBCB Number"=w423, "DofType"=w424) -> ("Offset"=w419:dbl)  [unwired: 8 in]
            n209 = Add(x=w420, y=w419) -> (x+y=w421:dbl)
            n210 = call "Slider Set Limit.vi"("DofType"=w424, "LBCB Number"=w423, "Value"=w421, "Index"=w422, "error in (no error)"=w418, "Lower/Upper"=Lower_Upper_Select."Upper") -> ("error out"=w417:errorcluster)  [unwired: 9 in]
          }
          frame 2 {
            n211 = call "Slider Set Limit.vi"("DofType"=w431, "LBCB Number"=w430, "Value"=w425, "Index"=w429, "error in (no error)"=w428, "Lower/Upper"=Lower_Upper_Select."Lower") -> ("error out"=w427:errorcluster)  [unwired: 9 in]
          }
          frame 3 {
            n212 = call "Slider Set Limit.vi"("DofType"=w438, "LBCB Number"=w437, "Value"=w432, "Index"=w436, "error in (no error)"=w435, "Lower/Upper"=Lower_Upper_Select."Upper") -> ("error out"=w434:errorcluster)  [unwired: 9 in]
          }
        }
        n213 = Enqueue Element(queue=w393, element=T4 {"Change State"=enum."Limits", "LBCB Number"=enum."LBCB1"}, error in (no error)=w391) -> (queue out=w392:refnum<queue>, error out=w390:errorcluster)  [unwired: 2 out]
        n214 = Enqueue Element(queue=w397, element=Slider_Messages."Update Display", error in (no error)=w390) -> (queue out=w396:refnum<queue>, error out=w395:errorcluster)  [unwired: 1 in, 1 out]
      }
      event Value Change {
        n215 = event-data() -> ("OldVal"=w455:string, "NewVal"=w454:string)  [unwired: 1 in, 3 out]
        n216 = local read "LBCB Number"() -> (w452:T2)
        n217 = local read "DofType"() -> (w453:T1)
        n218 = call "Limit Crossover Check.vi"("NewVal"=w454, "OldVal"=w455) -> ("Value"=w450:dbl, "Index"=w451:i32)
        n219 = case shown="0, Default" w451 {
          tunnel: w453 -> [w464 w473 w480 w487]
          tunnel: w452 -> [w463 w472 w479 w486]
          tunnel: w450 -> [w460 w469 w474 w481]
          tunnel: 2 ("Index") -> [w462 w471 w478 w485]
          tunnel: w448 -> [w458 w467 w477 w484]
          tunnel: [w457 w466 w476 w483] -> w441
          frame 0, Default {
            n220 = call "Slider Get Offset.vi"("Index"=w462, "LBCB Number"=w463, "DofType"=w464) -> ("Offset"=w459:dbl)  [unwired: 8 in]
            n221 = Add(x=w460, y=w459) -> (x+y=w461:dbl)
            n222 = call "Slider Set Limit.vi"("DofType"=w464, "LBCB Number"=w463, "Value"=w461, "Index"=w462, "error in (no error)"=w458, "Lower/Upper"=Lower_Upper_Select."Lower") -> ("error out"=w457:errorcluster)  [unwired: 9 in]
          }
          frame 1 {
            n223 = call "Slider Get Offset.vi"("Index"=w471, "LBCB Number"=w472, "DofType"=w473) -> ("Offset"=w468:dbl)  [unwired: 8 in]
            n224 = Add(x=w469, y=w468) -> (x+y=w470:dbl)
            n225 = call "Slider Set Limit.vi"("DofType"=w473, "LBCB Number"=w472, "Value"=w470, "Index"=w471, "error in (no error)"=w467, "Lower/Upper"=Lower_Upper_Select."Upper") -> ("error out"=w466:errorcluster)  [unwired: 9 in]
          }
          frame 2 {
            n226 = call "Slider Set Limit.vi"("DofType"=w480, "LBCB Number"=w479, "Value"=w474, "Index"=w478, "error in (no error)"=w477, "Lower/Upper"=Lower_Upper_Select."Lower") -> ("error out"=w476:errorcluster)  [unwired: 9 in]
          }
          frame 3 {
            n227 = call "Slider Set Limit.vi"("DofType"=w487, "LBCB Number"=w486, "Value"=w481, "Index"=w485, "error in (no error)"=w484, "Lower/Upper"=Lower_Upper_Select."Upper") -> ("error out"=w483:errorcluster)  [unwired: 9 in]
          }
        }
        n228 = Enqueue Element(queue=w442, element=T4 {"Change State"=enum."Limits", "LBCB Number"=enum."LBCB1"}, error in (no error)=w441) -> (queue out=w440:refnum<queue>, error out=w439:errorcluster)  [unwired: 2 out]
        n229 = Enqueue Element(queue=w446, element=Slider_Messages."Update Display", error in (no error)=w439) -> (queue out=w445:refnum<queue>, error out=w444:errorcluster)  [unwired: 1 in, 1 out]
      }
      event Value Change {
        n230 = event-data() -> ("OldVal"=w494:string, "NewVal"=w493:string)  [unwired: 1 in, 3 out]
        n231 = call "Limit Crossover Check.vi"("NewVal"=w493, "OldVal"=w494) -> ("Value"=w501:dbl, "Index"=w502:i32)
        n232 = local read "LBCB Number"() -> (w503:T2)
        n233 = local read "DofType"() -> (w504:T1)
        n234 = case shown="0, Default" w502 {
          tunnel: w504 -> [w513 w522 w529 w536]
          tunnel: w503 -> [w512 w521 w528 w535]
          tunnel: w501 -> [w509 w518 w523 w530]
          tunnel: 3 ("Index") -> [w511 w520 w527 w534]
          tunnel: w499 -> [w507 w516 w526 w533]
          tunnel: [w506 w515 w525 w532] -> w489
          frame 0, Default {
            n235 = call "Slider Get Offset.vi"("Index"=w511, "LBCB Number"=w512, "DofType"=w513) -> ("Offset"=w508:dbl)  [unwired: 8 in]
            n236 = Add(x=w509, y=w508) -> (x+y=w510:dbl)
            n237 = call "Slider Set Limit.vi"("DofType"=w513, "LBCB Number"=w512, "Value"=w510, "Index"=w511, "error in (no error)"=w507, "Lower/Upper"=Lower_Upper_Select."Lower") -> ("error out"=w506:errorcluster)  [unwired: 9 in]
          }
          frame 1 {
            n238 = call "Slider Get Offset.vi"("Index"=w520, "LBCB Number"=w521, "DofType"=w522) -> ("Offset"=w517:dbl)  [unwired: 8 in]
            n239 = Add(x=w518, y=w517) -> (x+y=w519:dbl)
            n240 = call "Slider Set Limit.vi"("DofType"=w522, "LBCB Number"=w521, "Value"=w519, "Index"=w520, "error in (no error)"=w516, "Lower/Upper"=Lower_Upper_Select."Upper") -> ("error out"=w515:errorcluster)  [unwired: 9 in]
          }
          frame 2 {
            n241 = call "Slider Set Limit.vi"("DofType"=w529, "LBCB Number"=w528, "Value"=w523, "Index"=w527, "error in (no error)"=w526, "Lower/Upper"=Lower_Upper_Select."Lower") -> ("error out"=w525:errorcluster)  [unwired: 9 in]
          }
          frame 3 {
            n242 = call "Slider Set Limit.vi"("DofType"=w536, "LBCB Number"=w535, "Value"=w530, "Index"=w534, "error in (no error)"=w533, "Lower/Upper"=Lower_Upper_Select."Upper") -> ("error out"=w532:errorcluster)  [unwired: 9 in]
          }
        }
        n243 = Enqueue Element(queue=w491, element=T4 {"Change State"=enum."Limits", "LBCB Number"=enum."LBCB1"}, error in (no error)=w489) -> (queue out=w490:refnum<queue>, error out=w488:errorcluster)  [unwired: 2 out]
        n244 = Enqueue Element(queue=w497, element=Slider_Messages."Update Display", error in (no error)=w488) -> (queue out=w496:refnum<queue>, error out=w495:errorcluster)  [unwired: 1 in, 1 out]
      }
      event Value Change {
        n245 = event-data() -> ("OldVal"=w553:string, "NewVal"=w552:string)  [unwired: 1 in, 3 out]
        n246 = local read "LBCB Number"() -> (w550:T2)
        n247 = call "Limit Crossover Check.vi"("NewVal"=w552, "OldVal"=w553) -> ("Value"=w548:dbl, "Index"=w549:i32)
        n248 = local read "DofType"() -> (w551:T1)
        n249 = case shown="0, Default" w549 {
          tunnel: w551 -> [w562 w571 w578 w585]
          tunnel: w550 -> [w561 w570 w577 w584]
          tunnel: w548 -> [w558 w567 w572 w579]
          tunnel: 4 ("Index") -> [w560 w569 w576 w583]
          tunnel: w546 -> [w556 w565 w575 w582]
          tunnel: [w555 w564 w574 w581] -> w538
          frame 0, Default {
            n250 = call "Slider Get Offset.vi"("Index"=w560, "LBCB Number"=w561, "DofType"=w562) -> ("Offset"=w557:dbl)  [unwired: 8 in]
            n251 = Add(x=w558, y=w557) -> (x+y=w559:dbl)
            n252 = call "Slider Set Limit.vi"("DofType"=w562, "LBCB Number"=w561, "Value"=w559, "Index"=w560, "error in (no error)"=w556, "Lower/Upper"=Lower_Upper_Select."Lower") -> ("error out"=w555:errorcluster)  [unwired: 9 in]
          }
          frame 1 {
            n253 = call "Slider Get Offset.vi"("Index"=w569, "LBCB Number"=w570, "DofType"=w571) -> ("Offset"=w566:dbl)  [unwired: 8 in]
            n254 = Add(x=w567, y=w566) -> (x+y=w568:dbl)
            n255 = call "Slider Set Limit.vi"("DofType"=w571, "LBCB Number"=w570, "Value"=w568, "Index"=w569, "error in (no error)"=w565, "Lower/Upper"=Lower_Upper_Select."Upper") -> ("error out"=w564:errorcluster)  [unwired: 9 in]
          }
          frame 2 {
            n256 = call "Slider Set Limit.vi"("DofType"=w578, "LBCB Number"=w577, "Value"=w572, "Index"=w576, "error in (no error)"=w575, "Lower/Upper"=Lower_Upper_Select."Lower") -> ("error out"=w574:errorcluster)  [unwired: 9 in]
          }
          frame 3 {
            n257 = call "Slider Set Limit.vi"("DofType"=w585, "LBCB Number"=w584, "Value"=w579, "Index"=w583, "error in (no error)"=w582, "Lower/Upper"=Lower_Upper_Select."Upper") -> ("error out"=w581:errorcluster)  [unwired: 9 in]
          }
        }
        n258 = Enqueue Element(queue=w540, element=T4 {"Change State"=enum."Limits", "LBCB Number"=enum."LBCB1"}, error in (no error)=w538) -> (queue out=w539:refnum<queue>, error out=w537:errorcluster)  [unwired: 2 out]
        n259 = Enqueue Element(queue=w544, element=Slider_Messages."Update Display", error in (no error)=w537) -> (queue out=w543:refnum<queue>, error out=w542:errorcluster)  [unwired: 1 in, 1 out]
      }
      event Value Change {
        n260 = event-data() -> ("OldVal"=w602:string, "NewVal"=w601:string)  [unwired: 1 in, 3 out]
        n261 = local read "LBCB Number"() -> (w599:T2)
        n262 = call "Limit Crossover Check.vi"("NewVal"=w601, "OldVal"=w602) -> ("Value"=w597:dbl, "Index"=w598:i32)
        n263 = local read "DofType"() -> (w600:T1)
        n264 = case shown="0, Default" w598 {
          tunnel: w600 -> [w611 w620 w627 w634]
          tunnel: w599 -> [w610 w619 w626 w633]
          tunnel: w597 -> [w607 w616 w621 w628]
          tunnel: 5 ("Index") -> [w609 w618 w625 w632]
          tunnel: w595 -> [w605 w614 w624 w631]
          tunnel: [w604 w613 w623 w630] -> w587
          frame 0, Default {
            n265 = call "Slider Get Offset.vi"("Index"=w609, "LBCB Number"=w610, "DofType"=w611) -> ("Offset"=w606:dbl)  [unwired: 8 in]
            n266 = Add(x=w607, y=w606) -> (x+y=w608:dbl)
            n267 = call "Slider Set Limit.vi"("DofType"=w611, "LBCB Number"=w610, "Value"=w608, "Index"=w609, "error in (no error)"=w605, "Lower/Upper"=Lower_Upper_Select."Lower") -> ("error out"=w604:errorcluster)  [unwired: 9 in]
          }
          frame 1 {
            n268 = call "Slider Get Offset.vi"("Index"=w618, "LBCB Number"=w619, "DofType"=w620) -> ("Offset"=w615:dbl)  [unwired: 8 in]
            n269 = Add(x=w616, y=w615) -> (x+y=w617:dbl)
            n270 = call "Slider Set Limit.vi"("DofType"=w620, "LBCB Number"=w619, "Value"=w617, "Index"=w618, "error in (no error)"=w614, "Lower/Upper"=Lower_Upper_Select."Upper") -> ("error out"=w613:errorcluster)  [unwired: 9 in]
          }
          frame 2 {
            n271 = call "Slider Set Limit.vi"("DofType"=w627, "LBCB Number"=w626, "Value"=w621, "Index"=w625, "error in (no error)"=w624, "Lower/Upper"=Lower_Upper_Select."Lower") -> ("error out"=w623:errorcluster)  [unwired: 9 in]
          }
          frame 3 {
            n272 = call "Slider Set Limit.vi"("DofType"=w634, "LBCB Number"=w633, "Value"=w628, "Index"=w632, "error in (no error)"=w631, "Lower/Upper"=Lower_Upper_Select."Upper") -> ("error out"=w630:errorcluster)  [unwired: 9 in]
          }
        }
        n273 = Enqueue Element(queue=w589, element=T4 {"Change State"=enum."Limits", "LBCB Number"=enum."LBCB1"}, error in (no error)=w587) -> (queue out=w588:refnum<queue>, error out=w586:errorcluster)  [unwired: 2 out]
        n274 = Enqueue Element(queue=w593, element=Slider_Messages."Update Display", error in (no error)=w586) -> (queue out=w592:refnum<queue>, error out=w591:errorcluster)  [unwired: 1 in, 1 out]
      }
    }
  }
  n275 = while {
    tunnel: w19 -> [w646]
    shift-right: [w643] -> _
    shift-left: w55 -> [w645]
    tunnel: [w638] -> w58
    shift-right: [w635] -> _
    shift-left: w12 -> [w637]
    stop <- w638 stop-if-true
    n276 = Dequeue Element(queue=w645, timeout in ms (-1)=2000, error in (no error)=w637) -> (queue out=w643:refnum<queue>, element=w641:T6, timed out?=w642:bool, error out=w636:errorcluster)
    n277 = Select(t=Slider_Messages."Nothing", s=w642, f=w641) -> (s? t:f=w639:T6)
    n278 = case shown="\"Update Display\"" w639 {
      tunnel: w646 -> [w679 _ _]
      tunnel: [_ TRUE _] -> w638
      tunnel: w636 -> [w651 w711 w713]
      tunnel: [w650 w711 w713] -> w635
      frame "Update Display" {
        n279 = local read "LBCB Number"() -> (w648:T2)
        n280 = local read "DofType"() -> (w653:T1)
        n281 = call "ReCheck Increment Limits.vi"("LBCB Number"=w648) -> ("error out"=w649:errorcluster)  [unwired: 10 in]
        n282 = local read "Limit Slider 1"() -> (w665:T3)
        n283 = local read "Limit Slider 2"() -> (w664:T3)
        n284 = local read "Limit Slider 3"() -> (w663:T3)
        n285 = local read "Limit Slider 4"() -> (w662:T3)
        n286 = local read "Limit Slider 5"() -> (w661:T3)
        n287 = local read "Limit Slider 6"() -> (w660:T3)
        n288 = call "FaultsList.vi"("error in (no error)"=w649, "Limits List Actions"=Faults_List_Actions."Get List") -> ("Fault List"=w654:T14[])  [unwired: 1 in, 8 out]
        n289 = call "Init Slider Boundaries.vi"("DofType"=w653) -> ("Unit Labels"=w657:string[], "Dof Labels"=w658:string[], "Boundaries"=w659:cluster{"[0]":dbl, "[1]":dbl}[])  [unwired: 8 in]
        n290 = call "Fault List 2 Array.vi"("Fault List"=w654, "LBCB Number"=w648, "DofType"=w653) -> ("Faults"=w655:bool[])  [unwired: 8 in]
        n291 = call "Fill Slider Values.vi"("LBCB Number"=w648, "DofType"=w653) -> ("Silder Values"=w652:T17)  [unwired: 9 in]
        n292 = Build Array(w665, w664, w663, w662, w661, w660) -> (w666:T3[])
        n293 = for {
          tunnel: w666 -> [w710] mode=indexing
          tunnel: [w709] -> w647 mode=indexing
          tunnel: w679 -> [w691] mode=indexing
          tunnel: w655 -> [w708] mode=indexing
          tunnel: w659 -> [w707] mode=indexing
          tunnel: w658 -> [w703] mode=indexing
          tunnel: w657 -> [w702] mode=indexing
          tunnel: w652 -> [w701] mode=indexing
          shift-right: [w681] -> w650
          shift-left: w651 -> [w682]
          n294 = Cluster To Array(cluster=w701) -> (array=w700:dbl[])
          n295 = Cluster To Array(cluster=w707) -> (array=w704:dbl[])
          n296 = Index Array(array=w700, index #1=0 ("index"), index #2=1 ("index"), index #3=2 ("index"), index #4=3 ("index"), index #5=4 ("index"), index #6=5 ("index")) -> (element #1=w686:dbl, element #2=w685:dbl, element #3=w688:dbl, element #4=w687:dbl, element #5=w694:dbl, element #6=w692:dbl)
          n297 = Index Array(array=w704, index #1=0 ("index"), index #2=1 ("index")) -> (element #1=w690:dbl, element #2=w689:dbl)
          n298 = Build Array(w688, w687, w686, w685) -> (w684:dbl[])
          n299 = Array To Cluster(array=w684) -> (cluster=w683:T19)
          n300 = Bundle By Name(cluster=w710, "DofLabel"=w703, "Units"=w702, "Local Lo 2"=w708, "Local Hi 1"=w686, "Global Actual 1"=w685, "Local Actual 1"=w688, "Global Lo 2"=w687, "Local Hi 2"=w694, "Local Actual 2"=w692, "DofLabel"=w683) -> (w709:T3)
          n301 = property class="Str"(reference=w691, error in=w682, "Scale.Minimum"=w690, "Scale.Maximum"=w689) -> (error out=w681:errorcluster)  [unwired: 1 out]
        }
        n302 = Index Array(array=w647, index #1=0 ("index"), index #2=1 ("index"), index #3=2 ("index"), index #4=3 ("index"), index #5=4 ("index"), index #6=5 ("index")) -> (element #1=w678:T3, element #2=w671:T3, element #3=w670:T3, element #4=w669:T3, element #5=w668:T3, element #6=w667:T3)
        n303 = disable-structure shown="Disabled" {
          disable-tunnel: w647 -> [w680 _]
          frame Disabled {
            n304 = call "Debug Limit Update.vi"("Slider Values"=w680) -> ()  [unwired: 11 in]
          }
          frame Enabled {
          }
        }
        n305 = local write "Limit Slider 1"(w678) -> ()
        n306 = local write "Limit Slider 2"(w671) -> ()
        n307 = local write "Limit Slider 3"(w670) -> ()
        n308 = local write "Limit Slider 4"(w669) -> ()
        n309 = local write "Limit Slider 5"(w668) -> ()
        n310 = local write "Limit Slider 6"(w667) -> ()
      }
      frame "Exit" {
      }
      frame "Nothing" {
      }
    }
  }
  n311 = Compound Arithmetic op=AND(w58, w57) -> (w56:bool)
  n312 = flat-sequence {
    tunnel: w56 -> [_]
    tunnel: w17 -> [w720]
    tunnel: w10 -> [w717]
    tunnel: w9 -> [w716]
    tunnel: [w714] -> w8
    frame #0 {
      n313 = control-ref of="This VI"() -> (w721:refnum<vi>)
      n314 = Release Queue(queue=w720, error in (no error)=w716) -> (error out=w715:errorcluster)  [unwired: 1 in, 2 out]
      n315 = local write "Ok"(FALSE ("Ok")) -> ()
      n316 = invoke class="VI" method="FP.Close"(reference=w721) -> ()  [unwired: 2 in, 3 out]
      n317 = Release Queue(queue=w717, error in (no error)=w715) -> (error out=w714:errorcluster)  [unwired: 1 in, 2 out]
      n318 = call "NoArgumentsLauncher.vi"("Application"=NoPanelAppTypes."Limits", "Application Launcher Actions"=Launcher_Actions."Stop") -> ()  [unwired: 8 in, 2 out]
    }
  }
  "error out" <- w8
